vi "read_all_waveforms.vi"(8 "error in (no error)":errorcluster, 10 "Small?":bool, 11 "Dust Event ID":i32) -> (0 "error out":errorcluster, 1 "Offset Array":dbl[](array[numeric]), 2 "dt":dbl, 3 "Waveform":T1)   [LabVIEW 2013]
uses:
  User Interface/Controls/Waveforms.ctl
  <vilib>/addons/h5labview/H5F_mode.ctl
  User Interface/Controls/Post_Signal.ctl
  User Interface/Controls/Role ID.ctl
  User Interface/Controls/Hardware ID.ctl
  <userlib>/_OpenG.lib/file/file.llb/File Exists - Scalar__ogtk.vi
  <vilib>/addons/h5labview/polymorph/H5A_read_var.vi
  <vilib>/addons/database/_DB Variant To Data/Database Variant To Data.xnode
  <vilib>/addons/h5labview/H5File.lvlib
  <vilib>/addons/h5labview/H5GroupObject.lvlib
  <vilib>/addons/h5labview/H5Attrib.lvlib
panel:
  out "Query Syntax":string
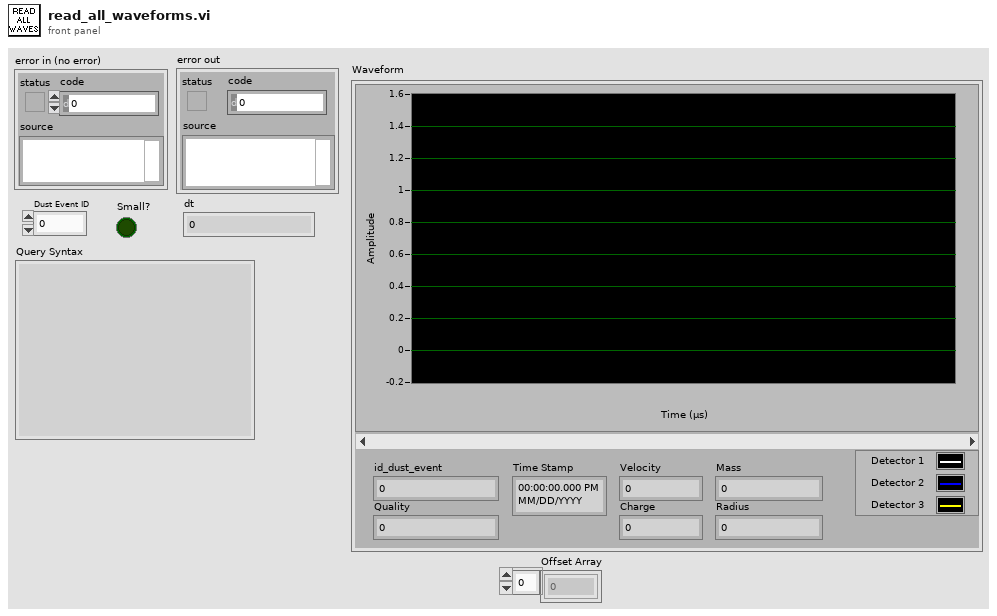
[diagram p1: front panel]
types:
  T1 = typedef "Waveforms.ctl" = cluster{"id_dust_event":u64, "Time Stamp":timestamp, "Velocity":dbl, "Mass":dbl, "Charge":dbl, "Radius":dbl, "Waveform Graph":sgl[][], "Quality":i32}
  T2 = typedef "H5File.lvlib/H5F_mode.ctl" = enum16{"read-only", "read-write", "overwrite", "create new", "open or create"}
  T3 = typedef "Role ID.ctl" = enum16{"First_Detector", "Second_Detector", "Third_Detector", "LeCroy_CH1", "LeCroy_CH2", "LeCroy_CH3", "LeCroy_CH4", "PSU", "DCS 1", "DCS 2"}
  T4 = typedef "Post_Signal.ctl" = cluster{"Integer Timestamp":i64, "Dust Event ID":i64, "Role ID":T3, "Data":sgl[], "Signal Length":i32, "dt":sgl, "Offset":dbl, "Hardware ID":T5}
  T5 = typedef "Hardware ID.ctl" = enum16{"Unknown", "CSA 1", "CSA 2", "CSA 3", "CSA 4", "CSA 5", "CSA 6", "DCS 1", "DCS 2"}
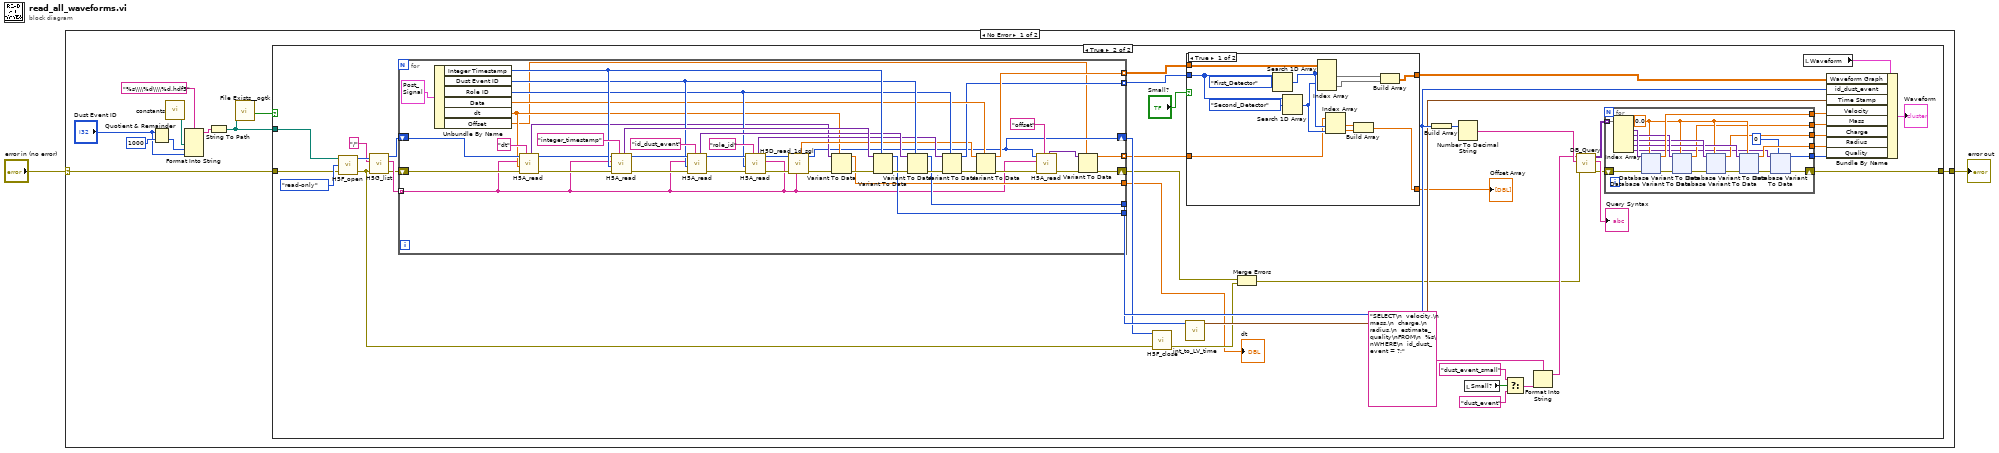
[diagram p0: block diagram]
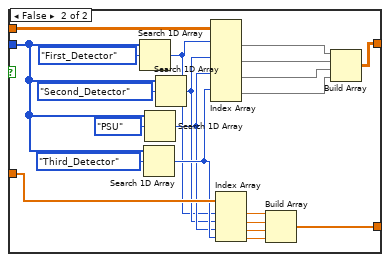
[diagram p3: hidden frame]
diagram:
  n1 = case shown="No Error" "error in (no error)" {
    selector: "error in (no error)" -> [w3 w313]
    tunnel: [w7 w313] -> w1
    frame No Error {
      n2 = Quotient & Remainder(x="Dust Event ID", y=1000) -> (floor(x/y)=w9:i32)  [unwired: 1 out]
      n3 = call "constants.vi"() -> ("file path for Processed Signal .hdf5 files"=w10:path)  [unwired: 3 in, 2 out]
      n4 = Format Into String(format string="%s\\\\%d\\\\%d.hdf5", w10, w9, "Dust Event ID") -> (resulting string=w4:string)  [unwired: 2 in, 1 out]
      n5 = String To Path(string=w4) -> (path=w5:path)
      n6 = call-poly <userlib>:"File Exists__ogtk.vi"("file path"=w5) -> ("exists"=w6:bool)  [unwired: 6 in, 1 out]
      n7 = case shown="True" w6 {
        tunnel: w5 -> [_ w55]
        tunnel: [w13 w53] -> w7
        tunnel: w3 -> [w13 w14]
        frame False {
        }
        frame True {
          n8 = call <vilib>:"H5F_open.vi"("error in (no error)"=w14, "mode"=H5F_mode."read-only", "path"=w55) -> ("error out"=w20:errorcluster, "ref"=w52:i32)  [unwired: 1 in]
          n9 = call <vilib>:"H5G_list.vi"("error in (no error)"=w20, "group"="/", "ref"=w52) -> ("error out"=w24:errorcluster, "names"=w28:string[], "ref out"=w25:i32)  [unwired: 1 in, 1 out]
          n10 = for {
            shift-right: [w271] -> w18
            shift-left: w24 -> [w285]
            shift-right: [w274] -> w26
            shift-left: w25 -> [w287]
            tunnel: w28 -> [w276] mode=indexing
            tunnel: [w291] -> w30 mode=indexing
            tunnel: [w292] -> w31 mode=indexing
            tunnel: [w289] -> w49
            tunnel: [w290] -> w32
            tunnel: [w280] -> w17
            tunnel: [w269] -> w16 mode=indexing
            n11 = Unbundle By Name(T4 {"Integer Timestamp"=0, "Dust Event ID"=0, "Role ID"=enum."First_Detector", "Data"=[], "Signal Length"=0, "dt"=0.0, "Offset"=0.0, "Hardware ID"=enum."CSA 1"} ("Post_Signal 2")) -> ("Integer Timestamp"=w310:i64, "Dust Event ID"=w304:i64, "Role ID"=w298:T3, "Data"=w295:sgl[], "dt"=w278:sgl, "Offset"=w270:dbl)
            n12 = call-poly <vilib>:"H5A_read.vi"("attrib_name"="dt", "error in (no error)"=w285, "default"=w278, "obj_name"=w276, "ref"=w287) -> ("error out"=w284:errorcluster, "ref out"=w286:i32, "value"=w281:variant)  [unwired: 2 in]
            n13 = call-poly <vilib>:"H5A_read.vi"("attrib_name"="integer_timestamp", "error in (no error)"=w284, "default"=w310, "obj_name"=w276, "ref"=w286) -> ("error out"=w306:errorcluster, "ref out"=w308:i32, "value"=w309:variant)  [unwired: 2 in]
            n14 = call-poly <vilib>:"H5A_read.vi"("attrib_name"="id_dust_event", "error in (no error)"=w306, "default"=w304, "obj_name"=w276, "ref"=w308) -> ("error out"=w302:errorcluster, "ref out"=w301:i32, "value"=w305:variant)  [unwired: 2 in]
            n15 = call-poly <vilib>:"H5A_read.vi"("attrib_name"="role_id", "error in (no error)"=w302, "default"=w298, "obj_name"=w276, "ref"=w301) -> ("error out"=w293:errorcluster, "ref out"=w294:i32, "value"=w299:variant)  [unwired: 2 in]
            n16 = call "H5D_read_1d_sgl.vi"("name"=w276, "error in (no error)"=w293, "ref"=w294) -> ("error out"=w283:errorcluster, "ref out"=w274:i32, "data"=w288:sgl[])  [unwired: 4 in]
            n17 = Variant To Data(error in=w283, type=w278, Variant=w281) -> (data=w280:sgl, error out=w282:errorcluster)
            n18 = Variant To Data(error in=w282, type=w310, Variant=w309) -> (data=w290:i64, error out=w303:errorcluster)
            n19 = Variant To Data(error in=w303, type=w304, Variant=w305) -> (data=w289:i64, error out=w297:errorcluster)
            n20 = Variant To Data(error in=w297, type=w298, Variant=w299) -> (data=w291:T3, error out=w296:errorcluster)
            n21 = Variant To Data(error in=w296, type=w295, Variant=w288) -> (data=w292:sgl[], error out=w277:errorcluster)
            n22 = call-poly <vilib>:"H5A_read.vi"("attrib_name"="offset", "error in (no error)"=w277, "obj_name"=w276, "ref"=w274) -> ("error out"=w272:errorcluster, "value"=w273:variant)  [unwired: 3 in, 1 out]
            n23 = Variant To Data(error in=w272, type=w270, Variant=w273) -> (data=w269:dbl, error out=w271:errorcluster)
          }
          "dt" <- w17
          n24 = call <vilib>:"H5F_close.vi"("error in (no error)"=w20, "ref"=w26) -> ("error out"=w21:errorcluster)  [unwired: 3 in]
          n25 = call "int_to_LV_time.vi"("Integer Timestamp"=w32) -> ("time stamp"=w33:timestamp)  [unwired: 8 in, 1 out]
          n26 = case shown="True" "Small?" {
            tunnel: w30 -> [w245 w261]
            tunnel: w31 -> [w244 w265]
            tunnel: [w242 w264] -> w22
            tunnel: w16 -> [w238 w257]
            tunnel: [w235 w248] -> w15
            frame True {
              n27 = Search 1D Array(1D array=w245, element=Role_ID."First_Detector") -> (index of element=w240:i32)  [unwired: 1 in]
              n28 = Search 1D Array(1D array=w245, element=Role_ID."Second_Detector") -> (index of element=w239:i32)  [unwired: 1 in]
              n29 = Index Array(array=w244, index (row) #1=w240, index (row) #2=w239) -> (element #1=w241:sgl[], element #2=w243:sgl[])  [unwired: 2 in]
              n30 = Index Array(array=w238, index #1=w240, index #2=w239) -> (element #1=w237:dbl, element #2=w236:dbl)
              n31 = Build Array(w237, w236) -> (w235:dbl[])
              n32 = Build Array(w241, w243) -> (w242:sgl[][])
            }
            frame False {
              n33 = Search 1D Array(1D array=w261, element=Role_ID."First_Detector") -> (index of element=w253:i32)  [unwired: 1 in]
              n34 = Search 1D Array(1D array=w261, element=Role_ID."Third_Detector") -> (index of element=w256:i32)  [unwired: 1 in]
              n35 = Search 1D Array(1D array=w261, element=Role_ID."PSU") -> (index of element=w255:i32)  [unwired: 1 in]
              n36 = Search 1D Array(1D array=w261, element=Role_ID."Second_Detector") -> (index of element=w254:i32)  [unwired: 1 in]
              n37 = Index Array(array=w265, index (row) #1=w253, index (row) #2=w254, index (row) #3=w255, index (row) #4=w256) -> (element #1=w259:sgl[], element #2=w258:sgl[], element #3=w263:sgl[], element #4=w260:sgl[])  [unwired: 4 in]
              n38 = Index Array(array=w257, index #1=w253, index #2=w254, index #3=w255, index #4=w256) -> (element #1=w252:dbl, element #2=w251:dbl, element #3=w250:dbl, element #4=w249:dbl)
              n39 = Build Array(w252, w251, w250, w249) -> (w248:dbl[])
              n40 = Build Array(w259, w258, w263, w260) -> (w264:sgl[][])
            }
          }
          "Offset Array" <- w15
          n41 = Merge Errors(w18, w21) -> (w19:errorcluster)
          n42 = Build Array(w49) -> (w50:i64[])
          n43 = Number To Decimal String(number=w50) -> (decimal integer string=w51:string[])  [unwired: 1 in]
          n44 = local read "Small?"() -> (w37:bool)
          n45 = Select(t="dust_event_small" ("resulting string"), s=w37, f="dust_event" ("resulting string")) -> (s? t:f=w36:string)
          n46 = Format Into String(format string="SELECT\n  velocity,\n  mass,\n  charge,\n  radius,\n  estimate_quality\nFROM\n  %s\nWHERE\n  id_dust_event = ?;" ("SQL query"), w36) -> (resulting string=w48:string)  [unwired: 2 in, 1 out]
          n47 = call "DB_Query.vi"("error in (no error)"=w19, "Parameters"=w51, "Parameterized Query"=w48) -> ("error out"=w45:errorcluster, "Query in Standard Format"=→"Query Syntax":string, "Results"=w46:variant[][])  [unwired: 6 in]
          n48 = for {
            tunnel: w46 -> [w73] mode=indexing
            shift-right: [w59] -> w53
            shift-left: w45 -> [w74]
            tunnel: [w70] -> w40
            tunnel: [w63] -> w41
            tunnel: [w62] -> w42
            tunnel: [w61] -> w43
            tunnel: [w56] -> w44
            w64 = 0.0 ("Velocity")
            n49 = Index Array(array=w73) -> (element #1=w72:variant, element #2=w69:variant, element #3=w67:variant, element #4=w65:variant, element #5=w58:variant)  [unwired: 5 in]
            n50 = xnode "Database Variant To Data"("database variant"=w72, "error in (no error)"=w74, "type"=w64) -> ("data"=w70:dbl, "error out"=w71:errorcluster)
            n51 = xnode "Database Variant To Data"("database variant"=w69, "error in (no error)"=w71, "type"=w64) -> ("data"=w63:dbl, "error out"=w68:errorcluster)
            n52 = xnode "Database Variant To Data"("database variant"=w67, "error in (no error)"=w68, "type"=w64) -> ("data"=w62:dbl, "error out"=w66:errorcluster)
            n53 = xnode "Database Variant To Data"("database variant"=w65, "error in (no error)"=w66, "type"=w64) -> ("data"=w61:dbl, "error out"=w60:errorcluster)
            n54 = xnode "Database Variant To Data"("database variant"=w58, "error in (no error)"=w60, "type"=i64 0 ("Dust Event ID")) -> ("data"=w56:i64, "error out"=w59:errorcluster)
          }
          n55 = local read "Waveform"() -> (w29:T1)
          n56 = Bundle By Name(cluster=w29, "Waveform Graph"=w22, "id_dust_event"=w49, "Time Stamp"=w33, "Velocity"=w40, "Mass"=w41, "Charge"=w42, "Radius"=w43, "Quality"=w44) -> (→"Waveform":T1)
        }
      }
    }
    frame Error {
    }
  }
  "error out" <- w1
